vi "Multirate Filter Simulation with Fixed-Point Inputs.vi"() -> ()   [LabVIEW 2023]
doc: "Demonstrates how to use the DFD FXP MRate Simulation VI to simulate fixed-point signals."
uses:
  <vilib>/addons/Digital Filter Design/Design.llb/DFD MRate Filter Design (Integer).vi
  <vilib>/addons/Digital Filter Design/FXPMRateSim.llb/DFD FXP MRate Simulation (DBL).vi
  <vilib>/addons/Digital Filter Design/FXPMRateSim.llb/DFD FXP MRate Postprocessing (I32, 1Ch).vi
  <vilib>/addons/Digital Filter Design/NI_DigFilterLicensed.lvlib
  <vilib>/Analysis/NI_AALBase.lvlib
panel:
  out "Error Message":string
  out "Filtering Results":dbl[](graph)
  in  "Output Word Length":i16=16
  in  "Coefficients Word Length":i16=16
  # "Select Help>>Show Context Help and move the cursor over the VI icon for more information."
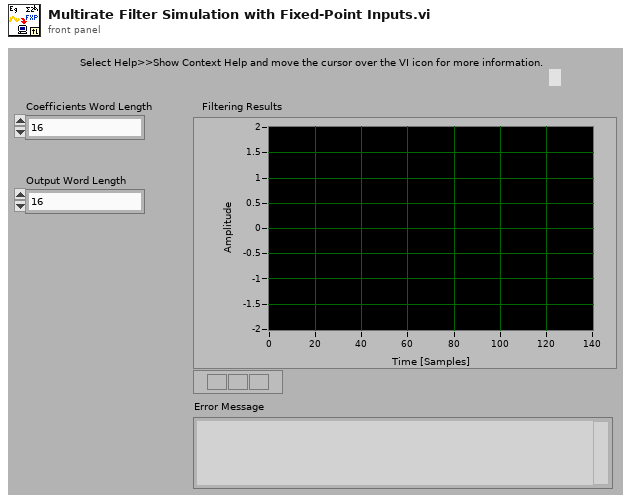
[diagram p1: front panel]
types:
  T1 = typedef "NI_DigFilterLicensed.lvlib/DFD Multirate Filter Obj.ctl" = cluster{"mMRate_Structure":enum16{"CIC", "FIR", "IIR", "Lattice"}, "mMRate_Mode":T2, "mMRate_Factor":i32, "mMRate_FIRParams":cluster{"mMRate_FIR_H":dbl[], "mMRate_FIR_IsNyquist?":bool, "mMRate_FIR_IsSymmetric?":bool}, "mMRate_CICParams":cluster{"mMRate_CIC_#Stage":i32, "mMRate_CIC_Lag":i32, "mMRate_CIC_Type":enum16{"Lowpass", "Highpass"}}, "mMRate_Order":i32, "mMRate_Version":string, "mMRate_Comments":string, "mMRate_RationalFactor":cluster{"mMRate_L":i32, "mMRate_M":i32}, "mMRate_Fs":dbl, "mMRate_Quantized?":bool, "mMRate_QFilterGain":dbl, "mMRate_CoefWl":i16, "mMRate_Scaling":cluster{"mMRate_ScaleByPowerOf2?":bool, "mMRate_ScaleType":T3}, "mMRate_InputWl":i16, "mMRate_OutputWl":i16, "mMRate_OutputMode":T4, "mMRate_MultMode":T5, "mMRate_BitPruning":bool, "mMRate_GainWl":i16, "mMRate_OutputFwl":i16, "mMRate_SumIwl":i16, "mMRate_InputIwl ":i16, "mMRate_SumWl":i16, "mMRate_CoefIwl":i16}
  T2 = typedef "NI_DigFilterLicensed.lvlib/DFD Multirate Mode.ctl" = i16
  T3 = typedef "NI_DigFilterLicensed.lvlib/DFD Coef Norm Type.ctl" = enum16{"No Norm", "Time Domain 1-Norm", "Time Domain 2-Norm", "Time Domain Inf-Norm"}
  T4 = typedef "NI_DigFilterLicensed.lvlib/DFD Round-off Mode.ctl" = enum16{"Nearest", "Truncation"}
  T5 = typedef "NI_DigFilterLicensed.lvlib/DFD FXP MRate Multiply Mode.ctl" = enum16{"Truncated", "Full"}
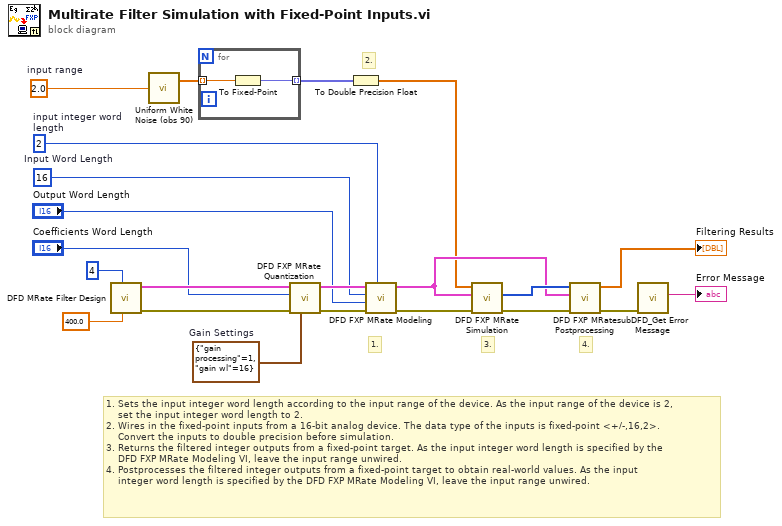
[diagram p0: block diagram]
diagram:
  w10 = i16 2  # input integer word length
  w12 = 2.0  # input range
  w11 = i16 16  # Input Word Length
  w19 = cluster{"gain processing":u16, "gain wl":i16} {"gain processing"=1, "gain wl"=16}  # Gain Settings
  # "3."
  # "4."
  # "2."
  # "1."
  # "1. Sets the input integer word length according to the input range of the device. As the input range of the device is 2,\n    set the input integer word length to 2.\n2. Wires in the fixed-point inputs from a 16-bit analog device. The data type of the inputs is fixed-point <+/-,16,2>. \n    Convert the inputs to double precision before simulation.\n3. Returns the filtered integer outputs from a fixed-point target. As the input integer word length is specified by the \n    DFD FXP MRate Modeling VI, leave the input range unwired.\n4. Postprocesses the filtered integer outputs from a fixed-point target to obtain real-world values. As the input \n    integer word length is specified by the DFD FXP MRate Modeling VI, leave the input range unwired."
  n1 = call-poly <vilib>:"DFD MRate Filter Design.vi"("fs in [Hz]"=400.0, "factor"=4) -> ("error out"=w4:errorcluster, "multirate filter out"=w5:T1)  [unwired: 6 in, 2 out]
  n2 = call <vilib>:"Uniform White Noise (obs 90).vi"("amplitude"=w12) -> ("uniform white noise"=w7:dbl[])  [unwired: 2 in, 1 out]
  n3 = for {
    tunnel: w7 -> [w24] mode=indexing
    tunnel: [w23] -> w6 mode=indexing
    n4 = To Fixed-Point(number=w24) -> (fixed-point=w23:fxp<+/-,16,2>)  [unwired: 1 out]
  }
  n5 = call <vilib>:"DFD FXP MRate Quantization.vi"("gain settings"=w19, "error in (no error)"=w4, "coefficients word length"="Coefficients Word Length", "multirate filter in"=w5) -> ("error out"=w17:errorcluster, "multirate filter out"=w18:T1)  [unwired: 2 in, 4 out]
  n6 = To Double Precision Float(number=w6) -> (double precision float=w2:dbl[])
  n7 = call <vilib>:"DFD FXP MRate Modeling.vi"("input integer word length"=w10, "error in (no error)"=w17, "output word length"="Output Word Length", "input word length"=w11, "multirate filter in"=w18) -> ("error out"=w15:errorcluster, "multirate filter out"=w9:T1)  [unwired: 3 in, 2 out]
  n8 = call-poly <vilib>:"DFD FXP MRate Simulation.vi"("error in (no error)"=w15, "multirate filter"=w9, "signal in"=w2) -> ("error out"=w14:errorcluster, "integer signal out"=w16:i32[])  [unwired: 2 in, 5 out]
  n9 = call-poly <vilib>:"DFD FXP MRate Postprocessing.vi"("error in (no error)"=w14, "multirate filter"=w9, "signal in"=w16) -> ("error out"=w13:errorcluster, "signal out"=→"Filtering Results":dbl[])  [unwired: 1 in, 6 out]
  n10 = call <vilib>:"subDFD_Get Error Message.vi"("error in (no error)"=w13) -> ("Error Message"=→"Error Message":string)  [unwired: 10 out]
